vi "A sample Text Slide.vi"   [LabVIEW 2010]
uses:
  SubVIs/LVPresent_Globals.vi
panel:
  # "This is a sample text slide"
  # "¥ Click on \"new slide\"\n¥ Select Text Slide\n¥ÊThis is just a labview front panel - compose at will\n\n¥ Movie slides - plave the movie in the movie folder - then it will do all the paths for you correctly when you select a Movie Template."
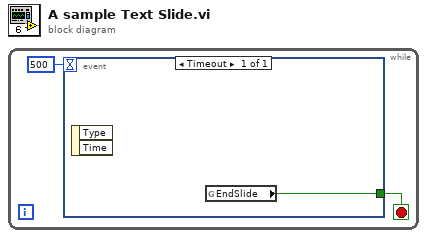
[diagram p0: block diagram]
diagram:
  n1 = while {
    stop <- w2 stop-if-true
    n2 = event shown="[0] Timeout" {
      selector: _ -> [_]
      dyn-events: _ -> [_]
      timeout: 500 -> [_]
      tunnel: [w3] -> w2
      event Timeout {
        n3 = event-data() -> ()  [unwired: 1 in, 2 out]
        n4 = global read "LVPresent_Globals.vi" "EndSlide"() -> (w3:bool)
      }
    }
  }
